vi "E13_Raíces.vi"() -> ()   [LabVIEW 2026]
panel:
  in  "Calcular":bool
  out "x/y 2":dbl
  out "x/y":dbl
  out "String":string
  in  "C":dbl
  in  "B":dbl
  in  "A":dbl
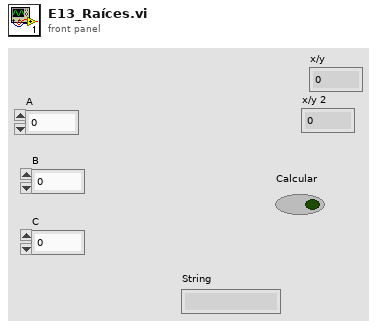
[diagram p1: front panel]
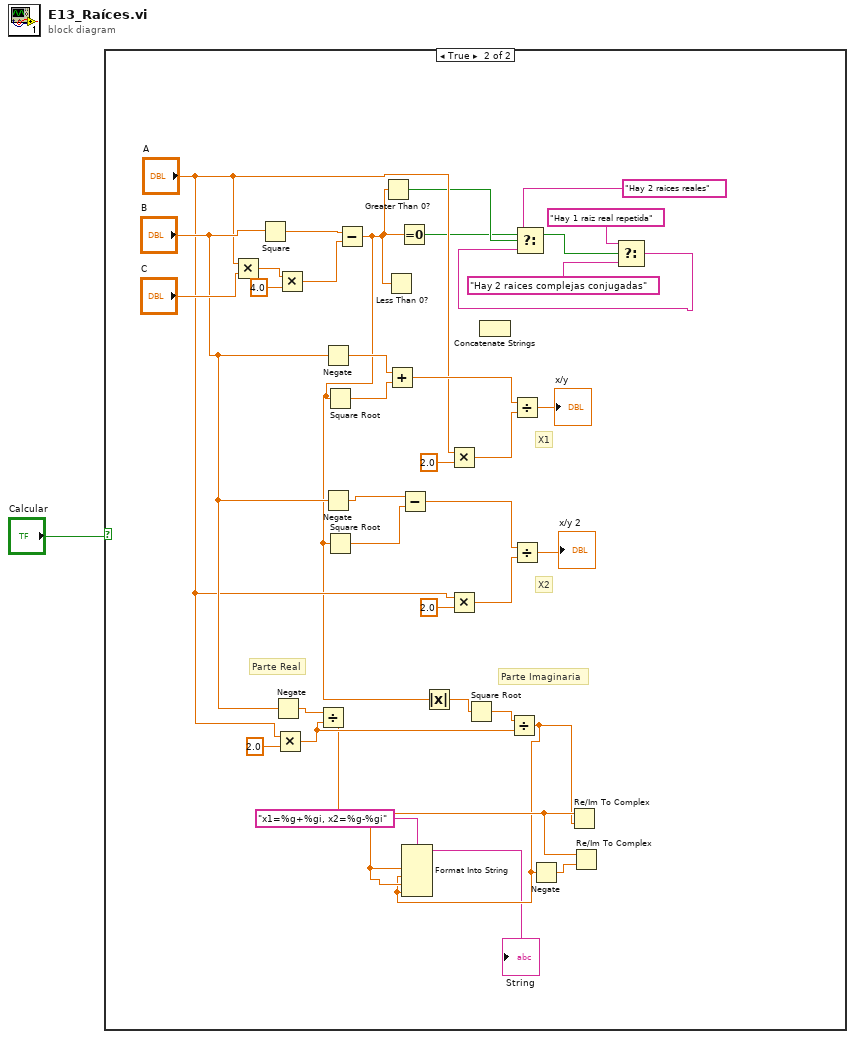
[diagram p0: block diagram]
diagram:
  n1 = case shown="True" "Calcular" {
    frame False {
    }
    frame True {
      # "Parte Imaginaria"
      # "Parte Real"
      # "X2"
      # "X1"
      n2 = Multiply(x="A", y="C") -> (x*y=w35:dbl)
      n3 = Square(x="B") -> (x^2=w37:dbl)
      n4 = Negate(x="B") -> (-x=w19:dbl)
      n5 = Multiply(x="A", y=2.0) -> (x*y=w15:dbl)
      n6 = Multiply(x=w35, y=4.0) -> (x*y=w36:dbl)
      n7 = Divide(x=w19, y=w15) -> (x/y=w13:dbl)
      n8 = Negate(x="B") -> (-x=w32:dbl)
      n9 = Negate(x="B") -> (-x=w25:dbl)
      n10 = Subtract(x=w37, y=w36) -> (x-y=w18:dbl)
      n11 = Square Root(x=w18) -> (sqrt(x)=w31:dbl)
      n12 = Square Root(x=w18) -> (sqrt(x)=w24:dbl)
      n13 = Greater Than 0?(x=w18) -> (x > 0?=w7:bool)
      n14 = Less Than 0?(x=w18) -> ()  [unwired: 1 out]
      n15 = Add(x=w32, y=w31) -> (x+y=w30:dbl)
      n16 = Equal To 0?(x=w18) -> (x = 0?=w5:bool)
      n17 = Subtract(x=w25, y=w24) -> (x-y=w23:dbl)
      n18 = Absolute Value(x=w18) -> (abs(x)=w17:dbl)
      n19 = Multiply(x="A", y=2.0) -> (x*y=w29:dbl)
      n20 = Multiply(x="A", y=2.0) -> (x*y=w27:dbl)
      n21 = Square Root(x=w17) -> (sqrt(x)=w16:dbl)
      n22 = Concatenate Strings() -> ()  [unwired: 2 in, 1 out]
      n23 = Divide(x=w16, y=w15) -> (x/y=w12:dbl)
      n24 = Format Into String(format string="x1=%g+%gi, x2=%g-%gi", w13, w12, w13, w12) -> (resulting string=→"String":string)  [unwired: 2 in, 1 out]
      n25 = Divide(x=w30, y=w29) -> (x/y=→"x/y":dbl)
      n26 = Divide(x=w23, y=w27) -> (x/y=→"x/y 2":dbl)
      n27 = Negate(x=w12) -> (-x=w14:dbl)
      n28 = Re/Im To Complex(1:w12, 2:w13) -> ()  [unwired: 1 out]
      n29 = Re/Im To Complex(1:w14, 2:w13) -> ()  [unwired: 1 out]
      n30 = Select(t="Hay 1 raiz real repetida", s=w5, f="Hay 2 raices complejas conjugadas") -> (s? t:f=w2:string)
      n31 = Select(t="Hay 2 raices reales", s=w7, f=w2) -> ()  [unwired: 1 out]
    }
  }
